vi "SubtractTime.vi"(1 "New Time Stamp":timestamp format="%<%I:%M:%S%4u %p\n%x>T", 2 "Old Time Stamp":timestamp format="%<%I:%M:%S%4u %p\n%x>T") -> (0 "Subtracted time":dbl)   [LabVIEW 2014]
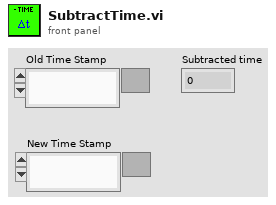
[diagram p1: front panel]
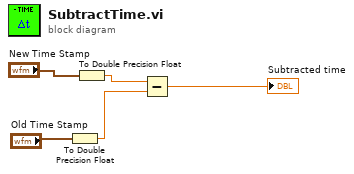
[diagram p0: block diagram]
diagram:
  n1 = To Double Precision Float(number="Old Time Stamp") -> (double precision float=w2:dbl)
  n2 = To Double Precision Float(number="New Time Stamp") -> (double precision float=w1:dbl)
  n3 = Subtract(x=w1, y=w2) -> (x-y=→"Subtracted time":dbl)
